vi "Add Entity.vi"(8 "error in (no error)":errorcluster, 10 "Conditum:Entity":refnum<class "Entity.lvclass">, 11 "Entity Collection in":refnum<class "Entity Collection.lvclass">) -> (0 "error out":errorcluster, 3 "Entity Collection out":refnum<class "Entity Collection.lvclass">)   [LabVIEW 2020, in "Conditu2.lvlib" / "Columns.lvlib" / "Entity Collection.lvclass"]
uses:
  Entity Collection.lvclass
  Entity/Entity.lvclass
  Entity Collection.lvclass/Entity Collection.ctl
  Entity/Entity.lvclass/Entity.ctl
  ID/ID.lvclass/ID.ctl
  ID/Get.vi
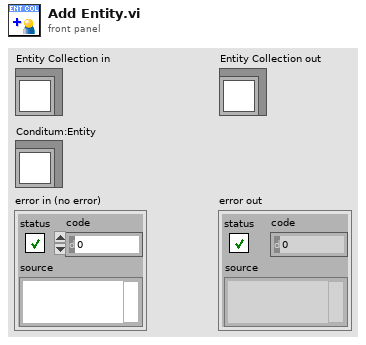
[diagram p1: front panel]
types:
  T1 = typedef "Conditu2.lvlib/Entity ID.ctl" = i64
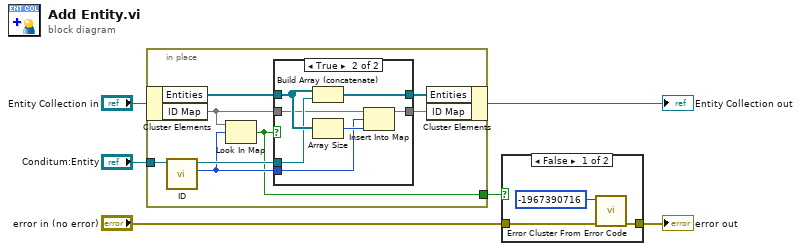
[diagram p0: block diagram]
diagram:
  n1 = in-place {
    in-place-border: "Conditum:Entity" -> [w14]
    in-place-border: [w7] -> w1
    n2 = in-place-cluster #1("Entity Collection in") -> ("Entities"=w13:refnum<class "Entity.lvclass">[], "ID Map"=w9:map{T1, i32})
    n3 = call "ID.vi"("Entity in"=w14) -> ("ID"=w8:T1, "Entity out"=w12:refnum<class "Entity.lvclass">)  [unwired: 9 in]
    n4 = Look In Map(map=w9, key=w8) -> (key not found?=w7:bool)  [unwired: 1 in, 1 out]
    n5 = case shown="True" w7 {
      tunnel: w13 -> [w16 w23]
      tunnel: w12 -> [_ w22]
      tunnel: [w16 w21] -> w11
      tunnel: [w15 w19] -> w10
      tunnel: w9 -> [w15 w18]
      tunnel: w8 -> [_ w17]
      frame False {
      }
      frame True {
        n6 = Build Array (concatenate)(w23, w22) -> (w21:refnum<class "Entity.lvclass">[])
        n7 = Array Size(array=w23) -> (size(s)=w20:i32)
        n8 = Insert Into Map(map in=w18, key=w17, value=w20) -> (map out=w19:map{T1, i32})  [unwired: 2 out]
      }
    }
    n9 = in-place-cluster #1("Entities"=w11, "ID Map"=w10) -> (→"Entity Collection out":refnum<class "Entity Collection.lvclass">)
  }
  n10 = case shown="False" w1 {
    tunnel: "error in (no error)" -> [w26 w27]
    tunnel: [w25 w27] -> w2
    frame False {
      n11 = call <vilib>:"Error Cluster From Error Code.vi"("error in (no error)"=w26, "error code (0)"=-1967390716) -> ("error out"=w25:errorcluster)  [unwired: 7 in]
    }
    frame True {
    }
  }
  "error out" <- w2
